vi "Main.vi"() -> ()   [LabVIEW 2020, in "Application.lvlib"]
uses:
  Application.lvlib
  Data Manager/Name--cluster.ctl
  Data Manager/Profile--cluster.ctl
  Strava/Strava curl/Strava curl.lvclass
  Data Manager/Data Manager.lvclass
  Globals.vi
  <userlib>/FTools/JSON Pretty Printer/JSON Pretty Printer.lvlib
  Twitter/Twitter.lvclass
  Visualisation/Visualisation.lvclass
panel:
  out "Status":string
  out "Errors":errorcluster[](array[cluster])
  in  "Tab":T1(tab)
  in  "Date for Daily Gains":timestamp format="%<%x %.3X>T"
  in  "Download from Strava":bool
  in  "Strava":T2={"Club ID"="RockCrusaders", "page"="1", "per_page"="200", "Authentication Token"=""}
  in  "Update Athlete":bool
  out "Athlete Profile Map":map{T3, T4}(c390)
  in  "Load Members":bool
  in  "path to PNG file":path=path "C:/Users/User/Documents/GitHub/StravaLabVIEWTwitter/Exports/To Publish.png"
  in  "Tweet":string="\n\n@RockcrusadersO #Strava #Run #Walk #Ride #FebruaryChallenge #TweetBot"
  in  "Tweet with Image":bool
  in  "Preview":bool
  out "History":string[][](table)
  in  "SQL":string
  out "Return":string[][](table)
  in  "Run SQL":bool
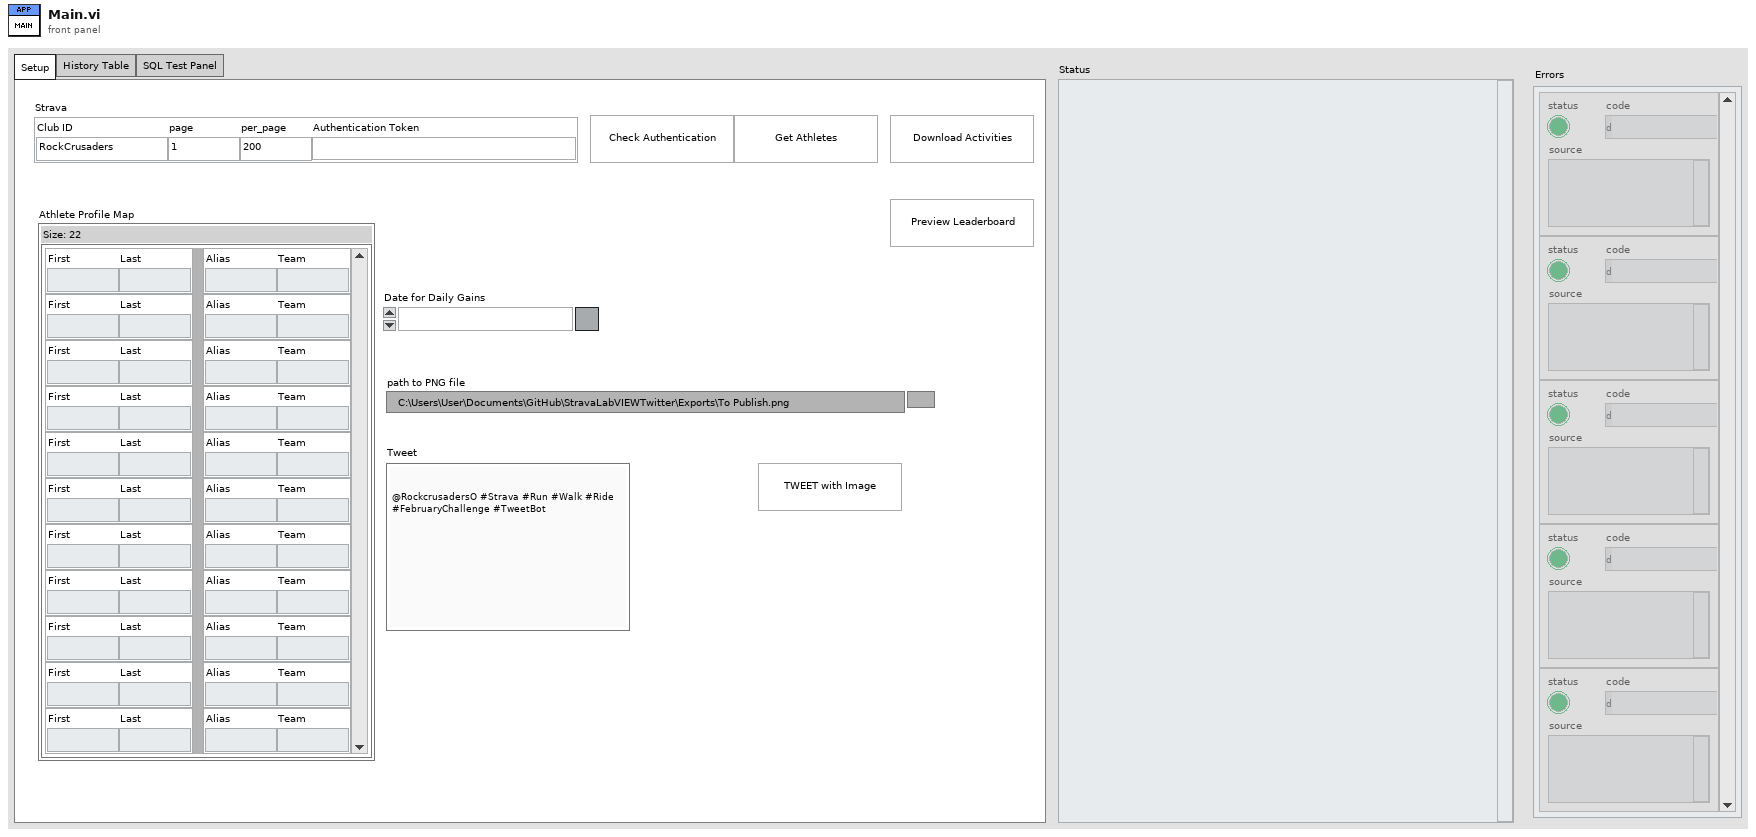
[diagram p1: front panel]
types:
  T1 = enum32{"Setup", "History Table", "SQL Test Panel"}
  T2 = cluster{"Club ID":string, "page":string, "per_page":string, "Authentication Token":string}
  T3 = typedef "Data Manager.lvclass/Name--cluster.ctl" = cluster{"First":string, "Last":string}
  T4 = typedef "Data Manager.lvclass/Profile--cluster.ctl" = cluster{"Alias":string, "Team":string}
  T5 = enum32{"Invalid", "Standard", "Closed", "Hidden", "Minimized", "Maximized"}
  T6 = enum32{"invalid app kind", "Development System", "Run Time System", "Student Edition", "Embedded LabVIEW", "Evaluation", "Custom"}
  T7 = cluster{"Record Headers":string[], "All Records":string[][]}
  T8 = cluster{"Core":cluster{"Current VI Reference":refnum<vi>, "Close Panel on Exit?":bool}, "Errors":errorcluster[], "Strava":refnum<class "Strava curl.lvclass">, "Data Manager":refnum<class "Data Manager.lvclass">}
  T9 = cluster{"Current VI Reference":refnum<vi>, "Close Panel on Exit?":bool}
  T10 = typedef "Data Manager.lvclass/Strava JSON for Club Activities--cluster.ctl" = cluster{"athlete":cluster{"firstname":string, "lastname":string}, "type":string, "distance":dbl, "moving_time":dbl, "elapsed_time":dbl, "total_elevation_gain":dbl}
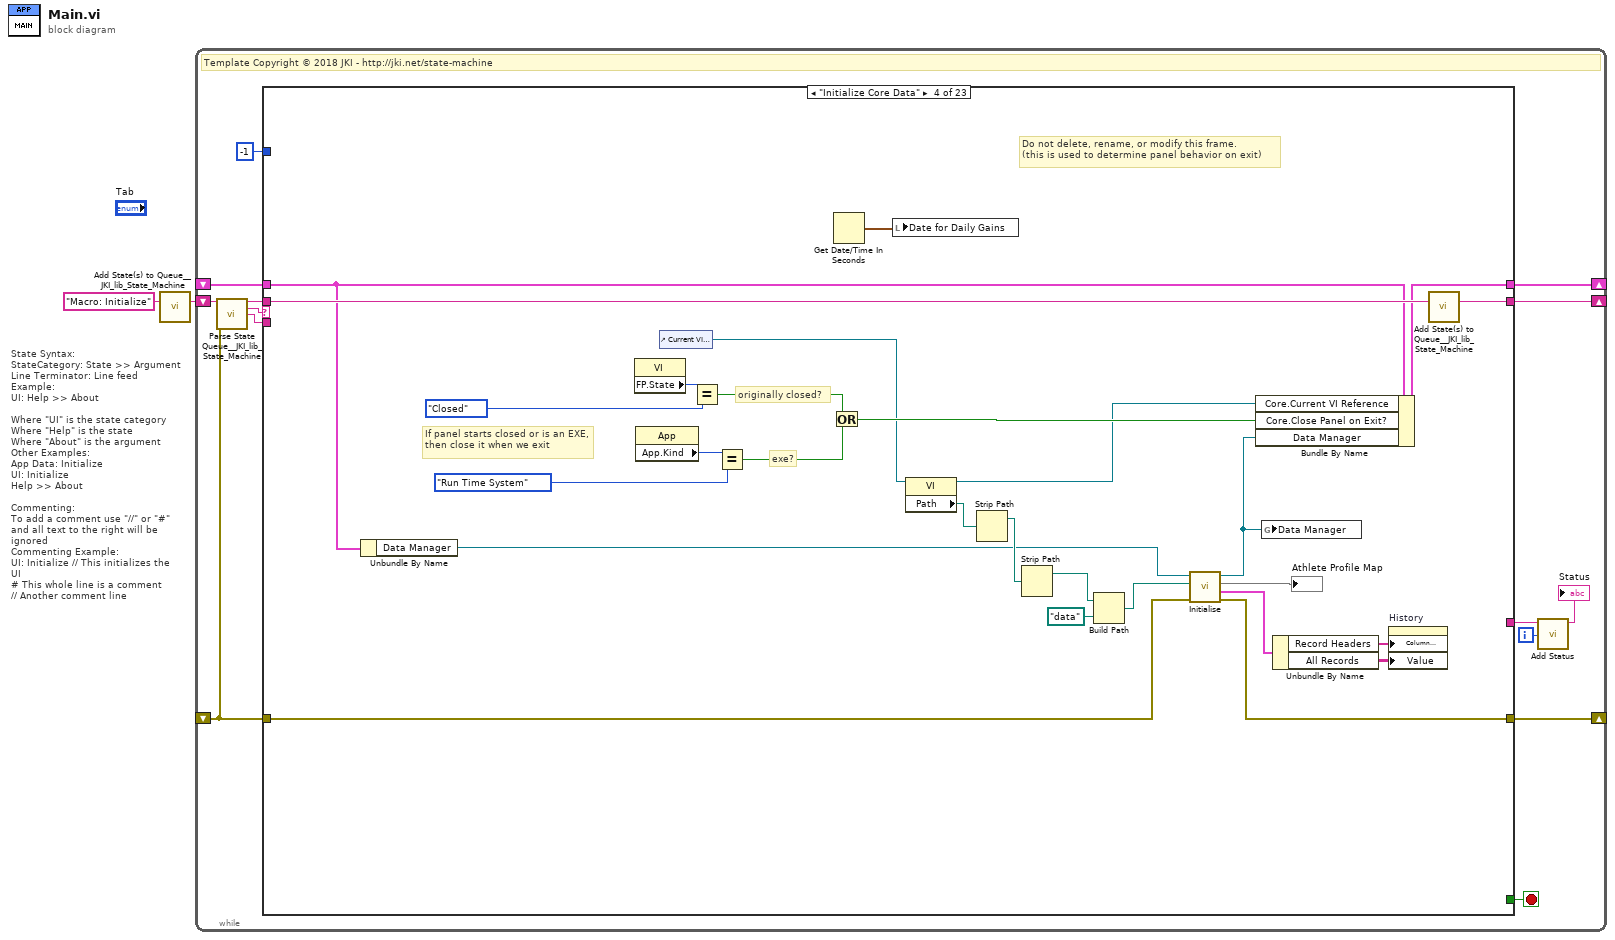
[diagram p0: block diagram]
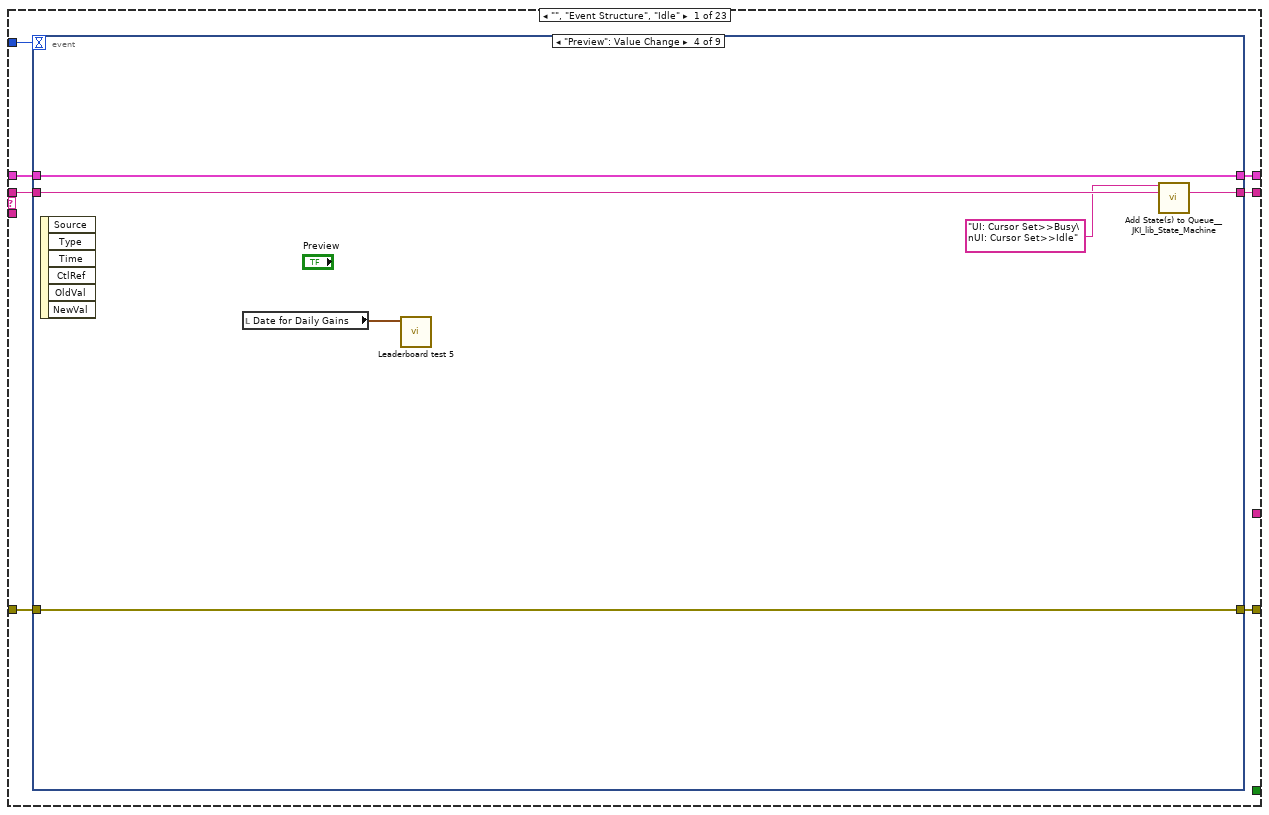
[diagram p2: hidden frame]
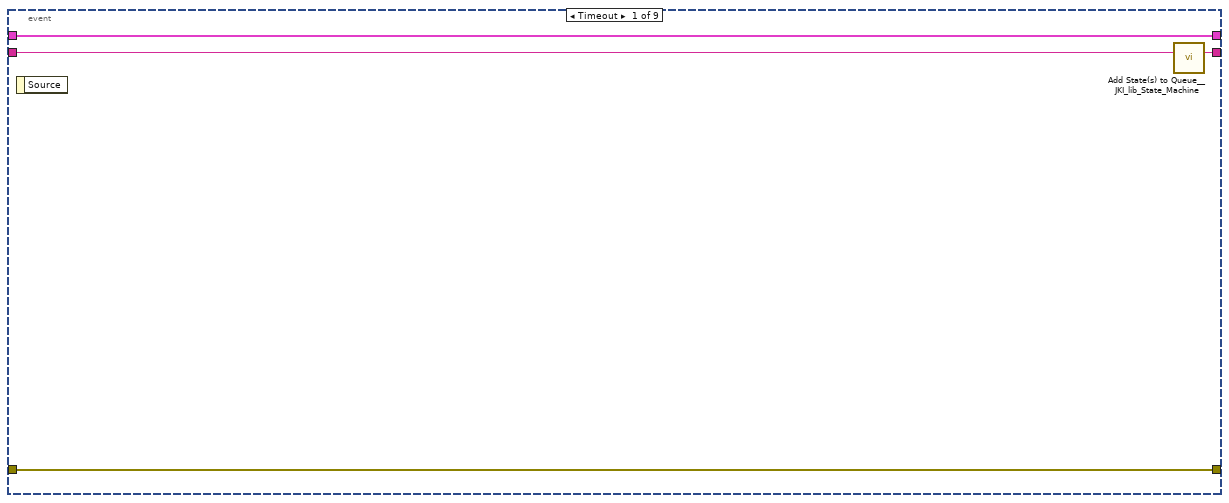
[diagram p3: hidden frame]
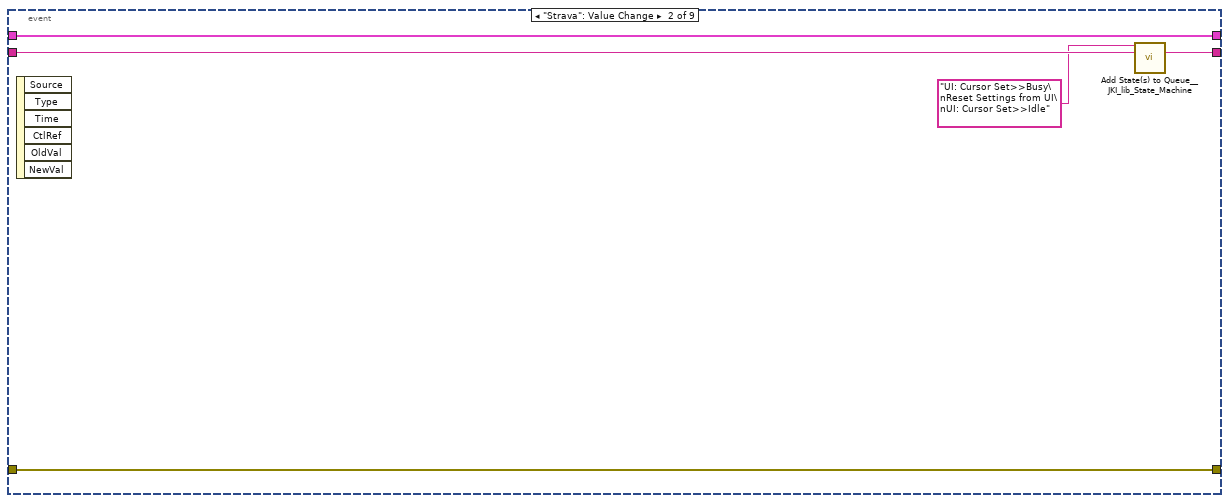
[diagram p4: hidden frame]
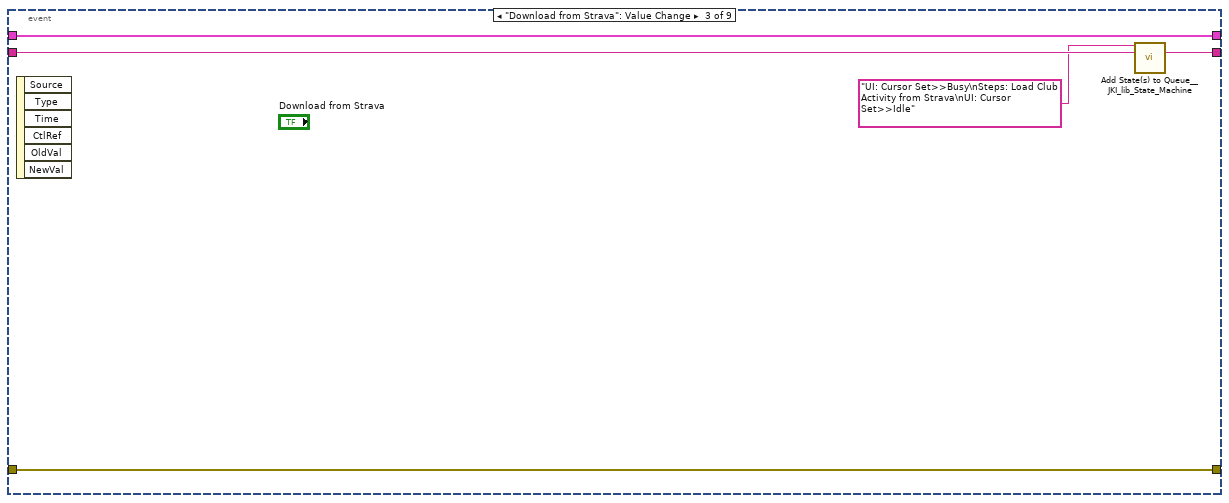
[diagram p5: hidden frame]
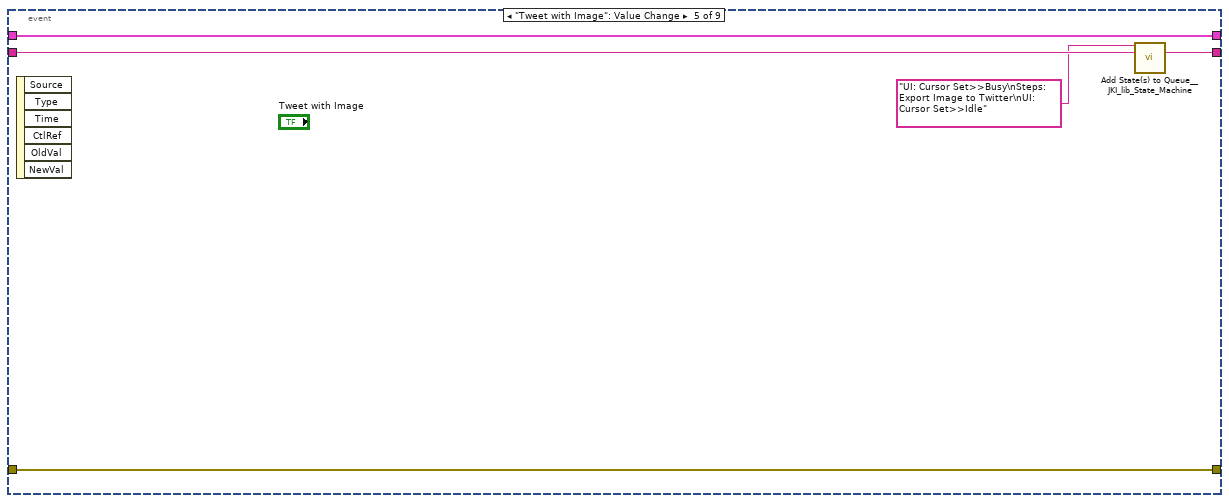
[diagram p6: hidden frame]
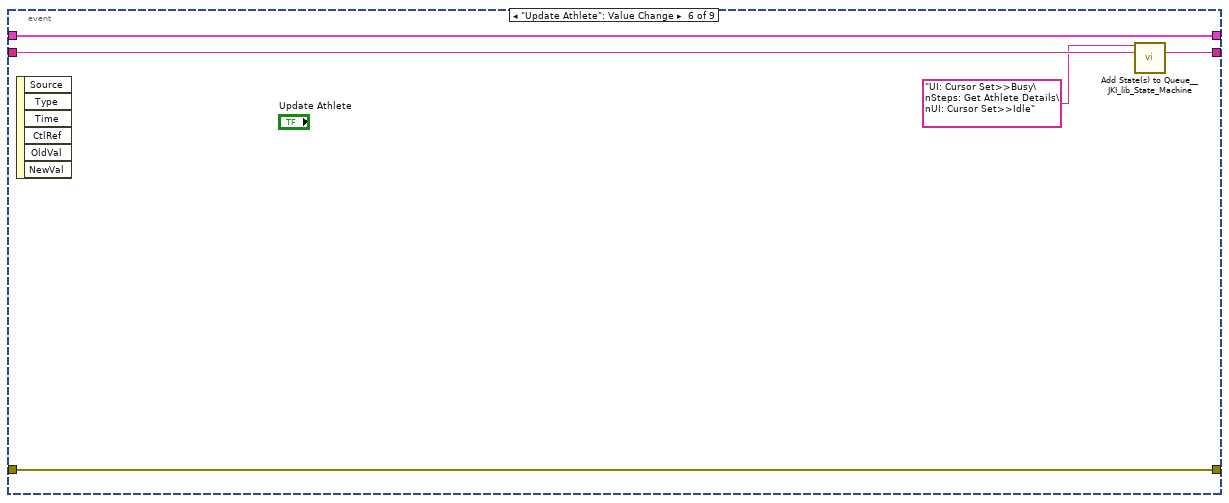
[diagram p7: hidden frame]
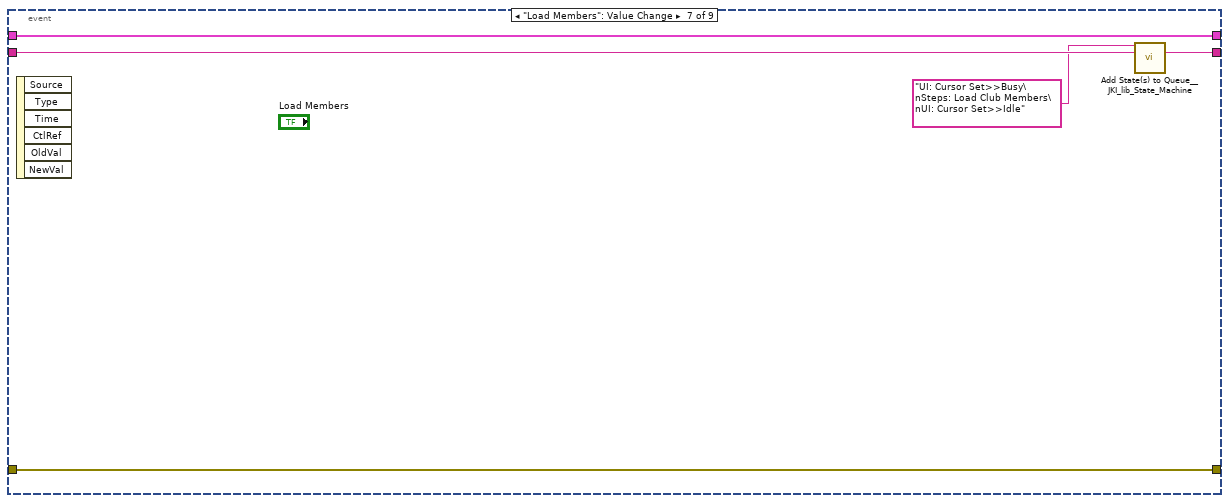
[diagram p8: hidden frame]
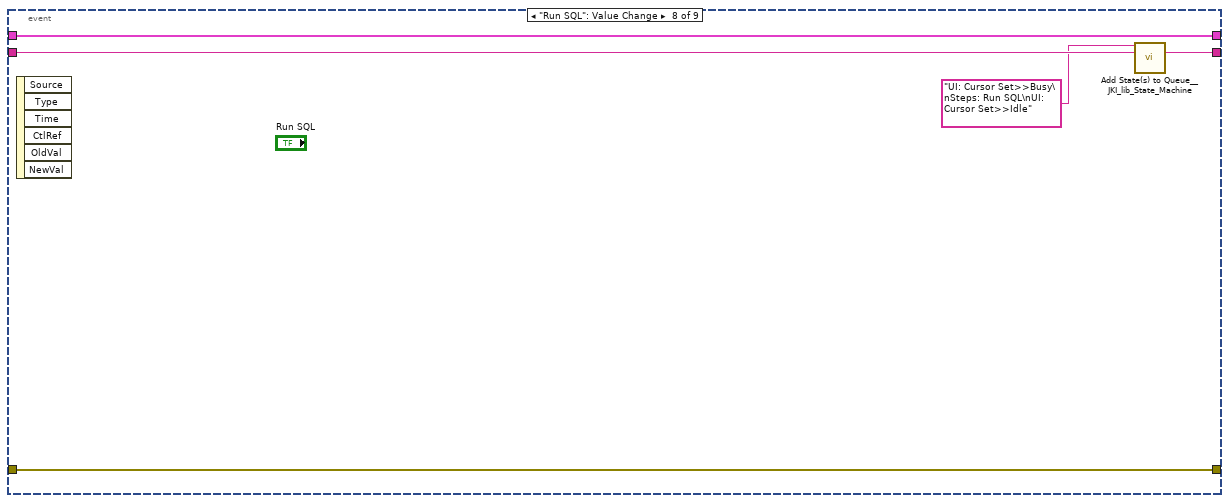
[diagram p9: hidden frame]
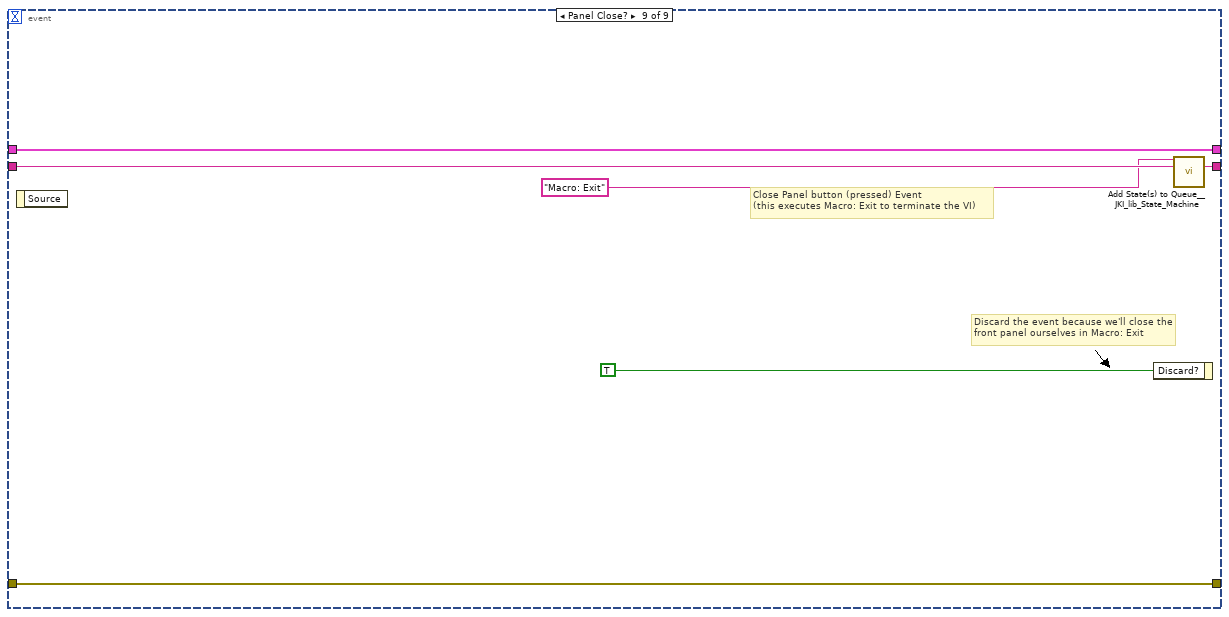
[diagram p10: hidden frame]
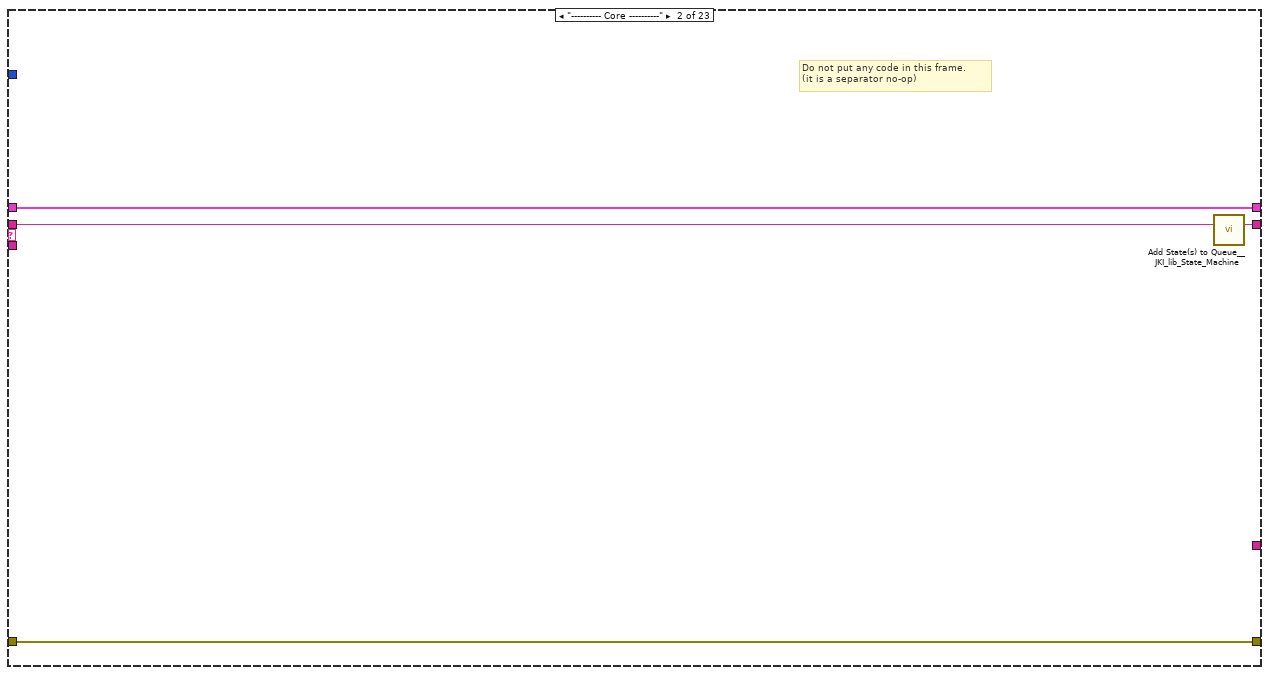
[diagram p11: hidden frame]
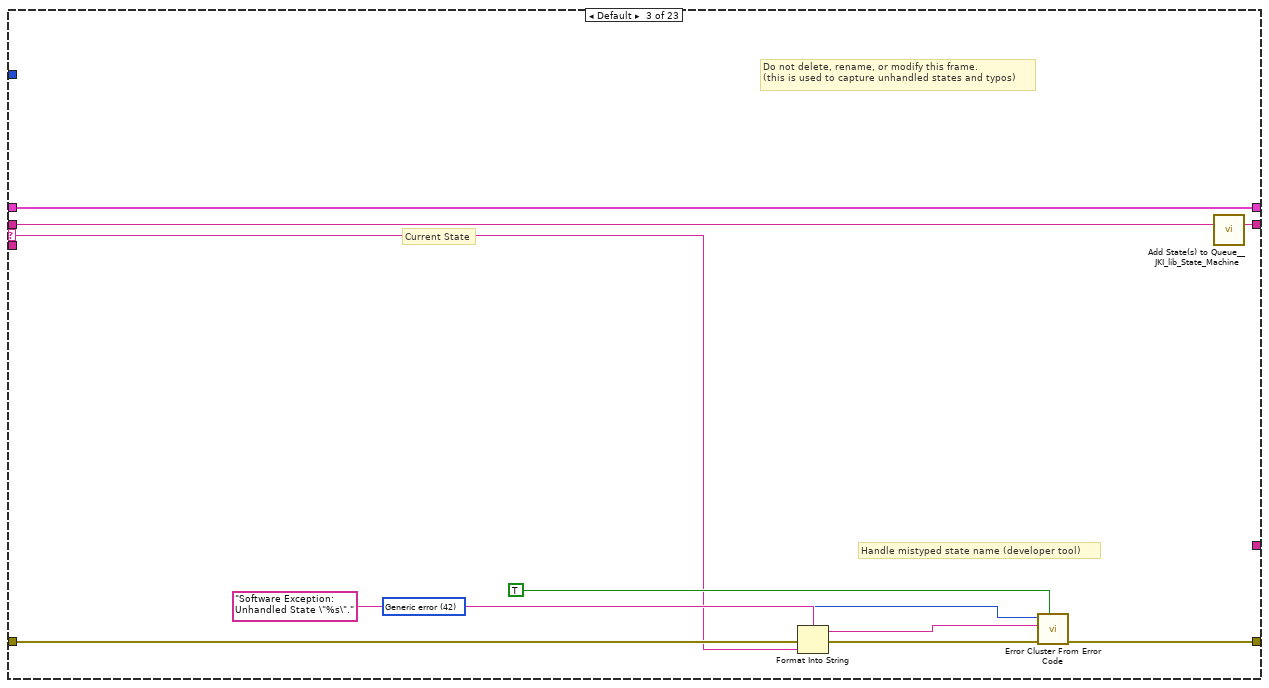
[diagram p12: hidden frame]
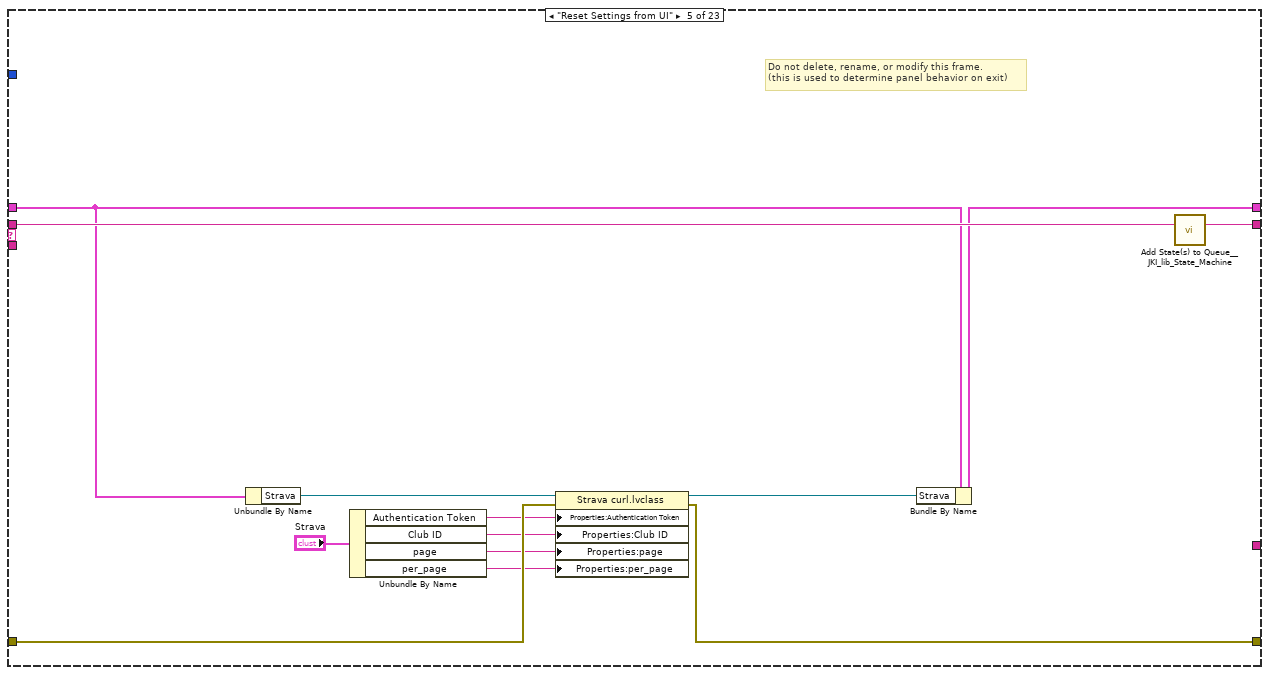
[diagram p13: hidden frame]
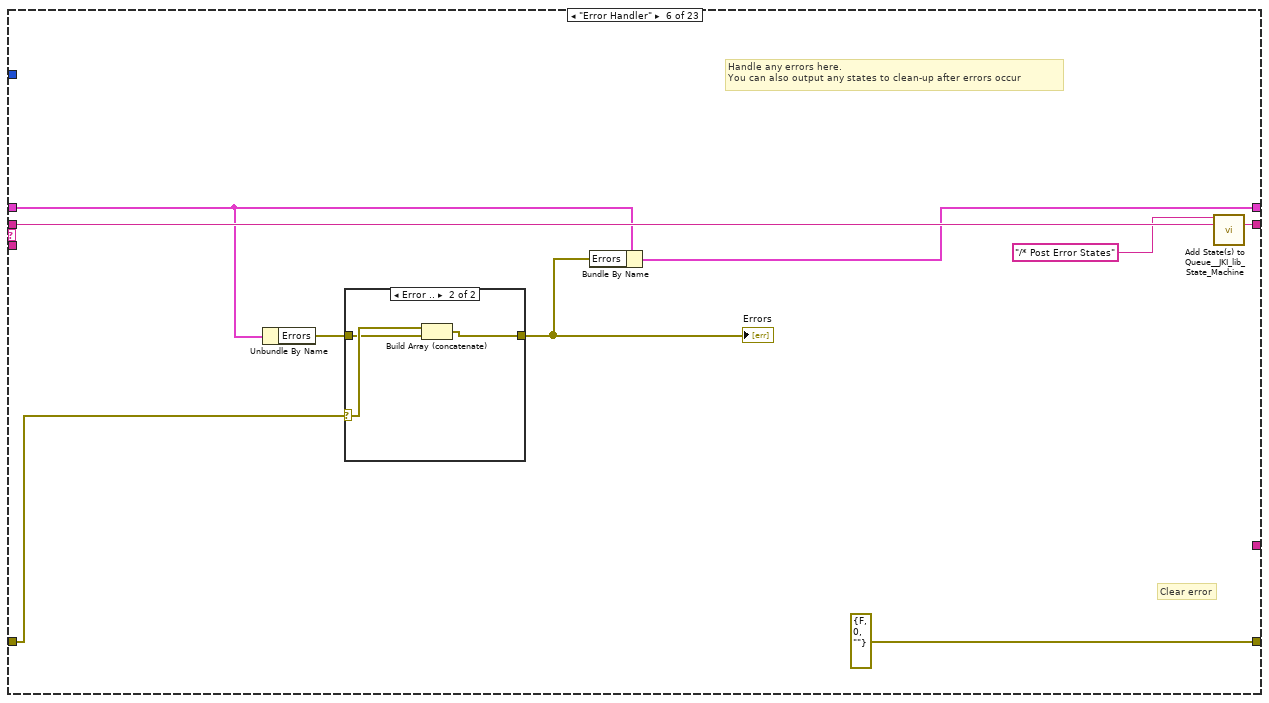
[diagram p14: hidden frame]
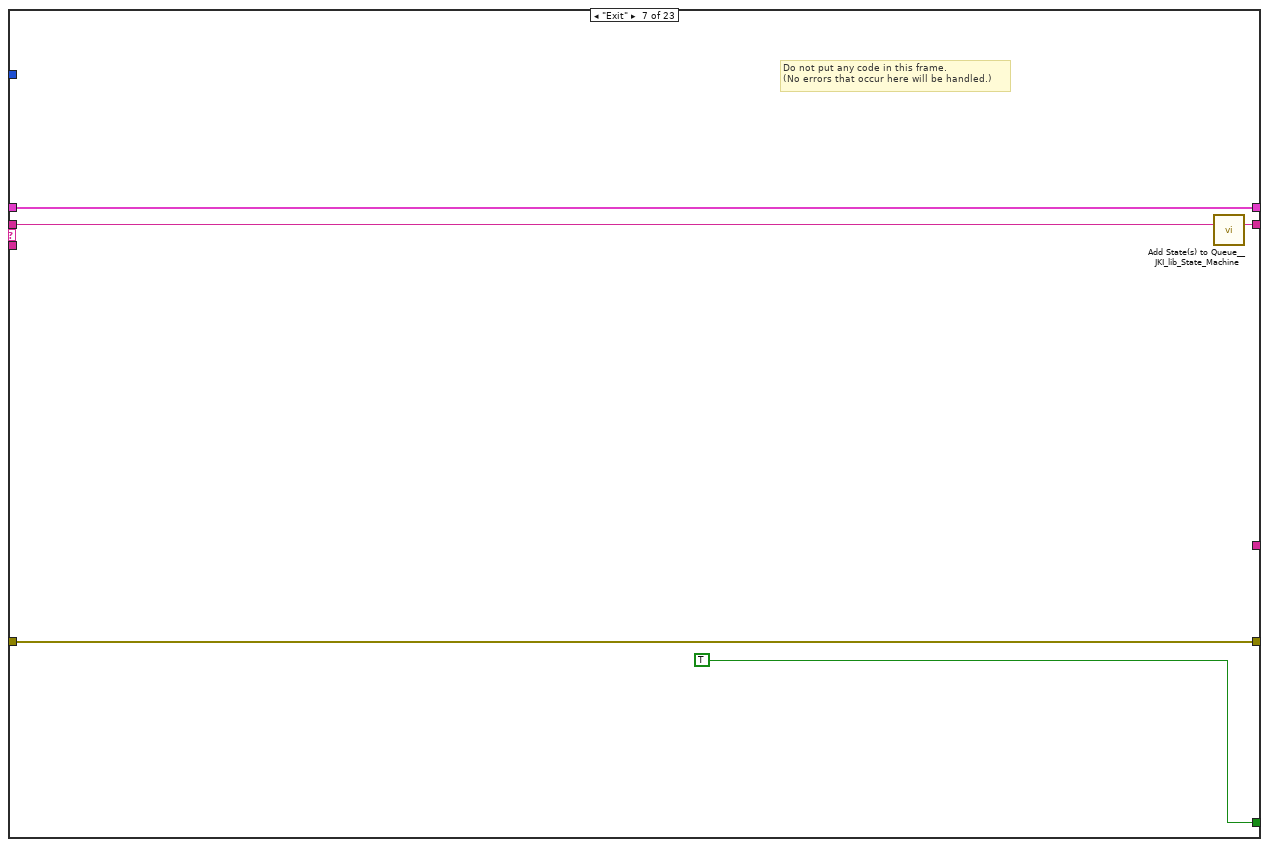
[diagram p16: hidden frame]
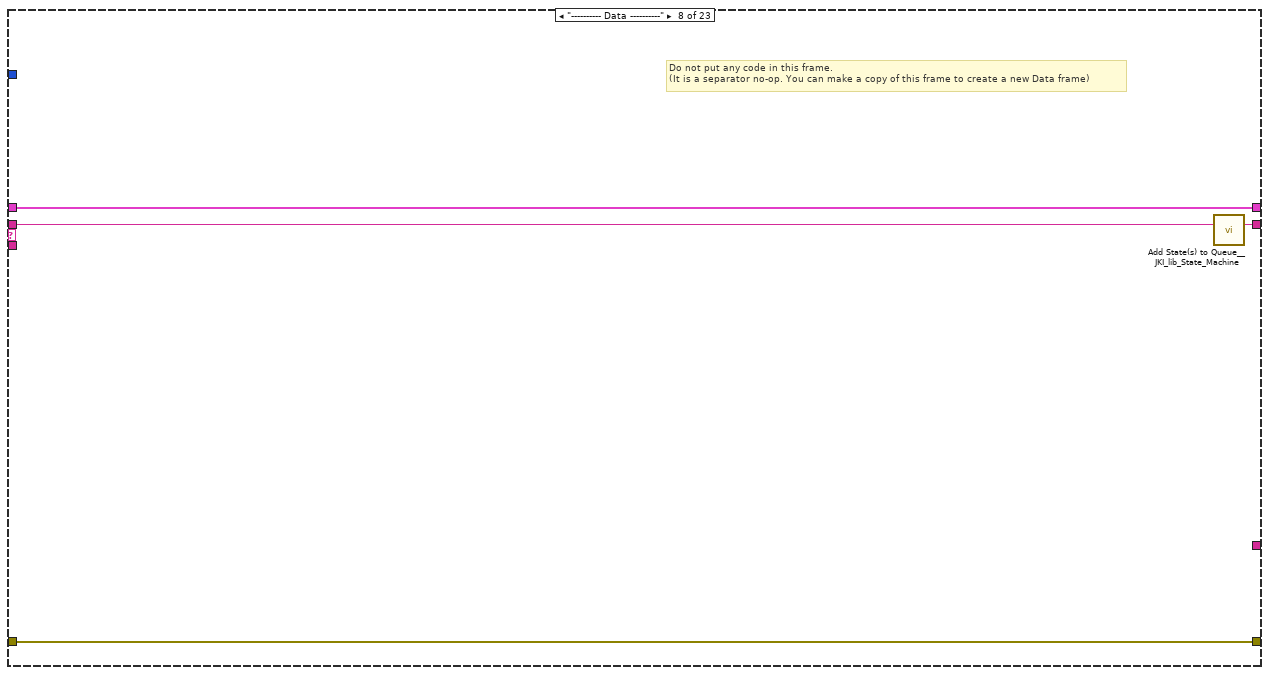
[diagram p17: hidden frame]
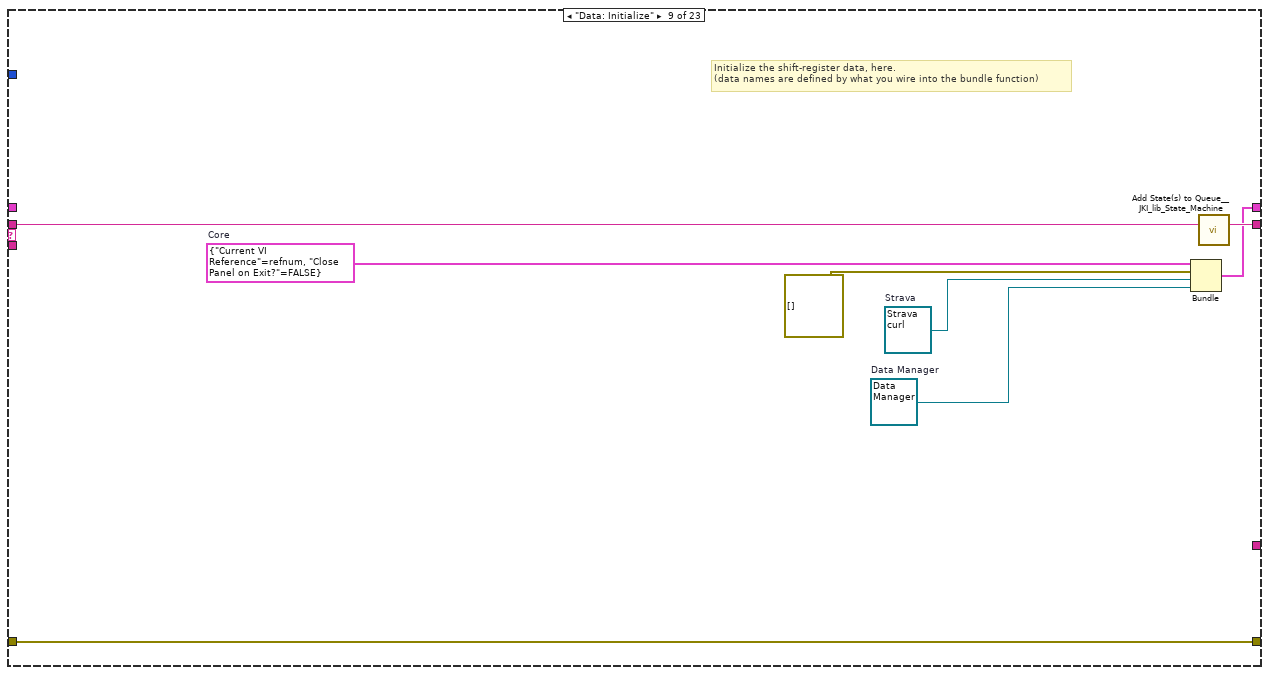
[diagram p18: hidden frame]
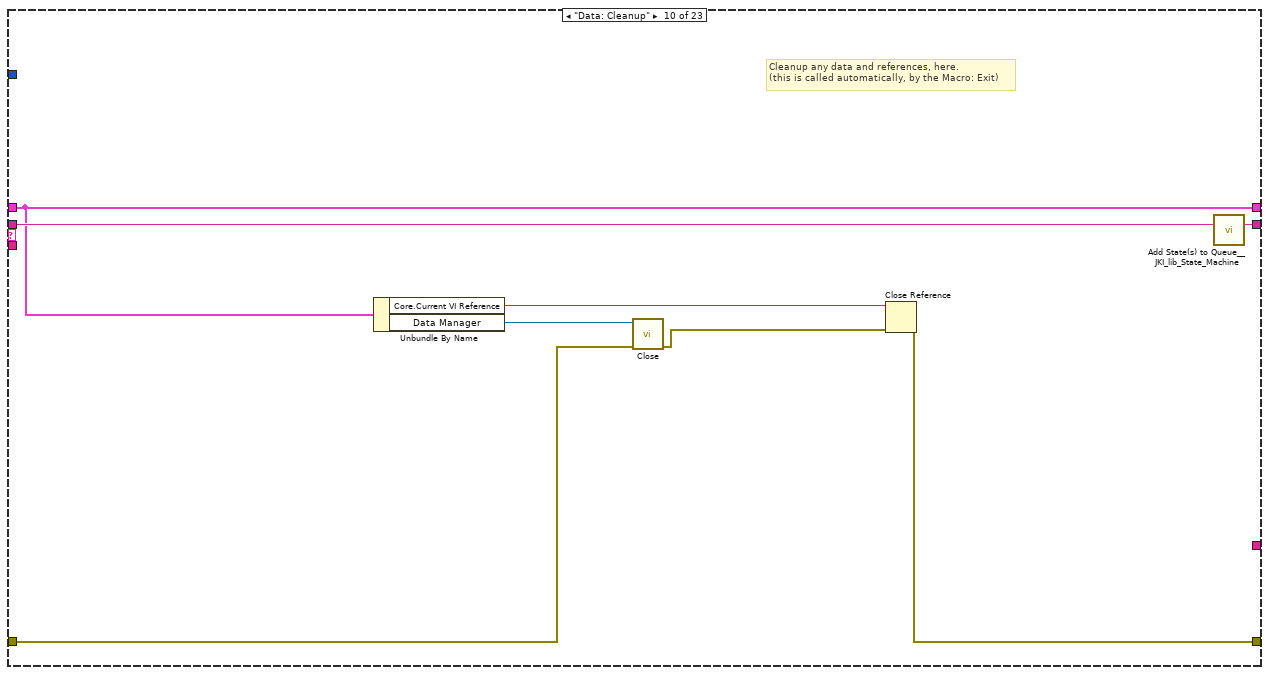
[diagram p19: hidden frame]
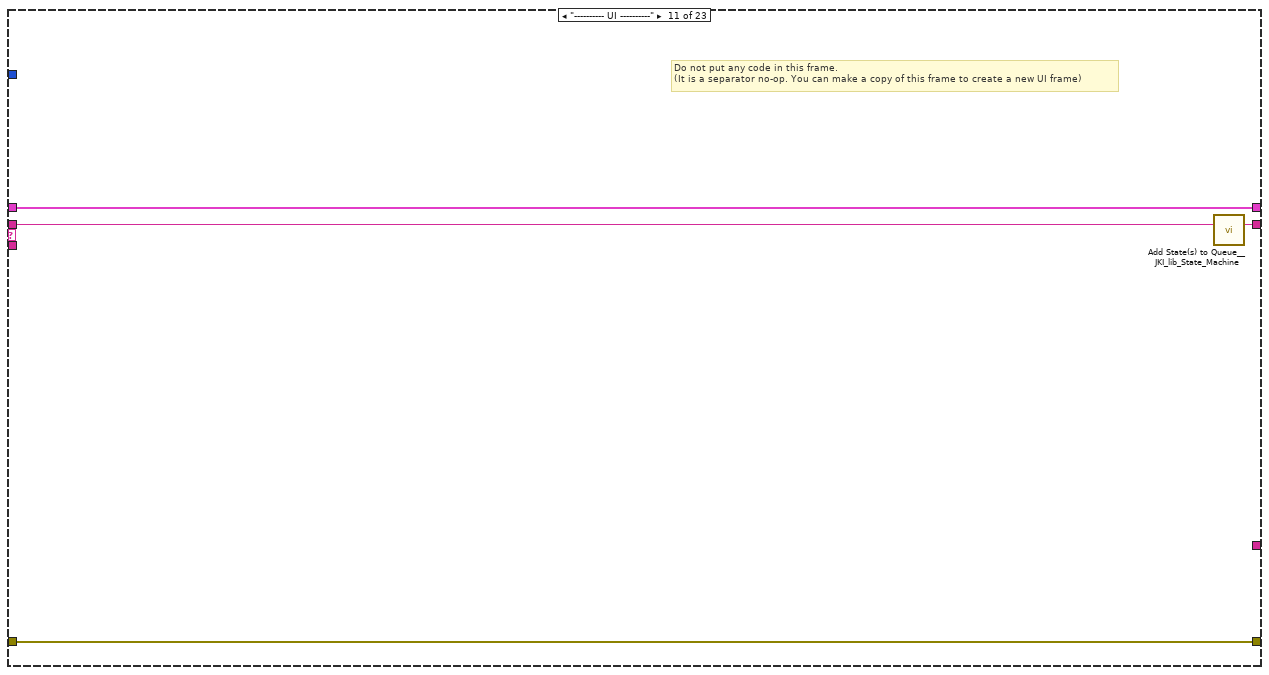
[diagram p20: hidden frame]
diagram:
  # "State Syntax:\nStateCategory: State >> Argument\nLine Terminator: Line feed\nExample:\nUI: Help >> About\n\nWhere \"UI\" is the state category\nWhere \"Help\" is the state\nWhere \"About\" is the argument\nOther Examples:\nApp Data: Initialize\nUI: Initialize\nHelp >> About\n\nCommenting:\nTo add a comment use \"//\" or \"#\" and all text to the right will be ignored\nCommenting Example:\nUI: Initialize // This initializes the UI\n# This whole line is a comment\n// Another comment line"
  n1 = call <vilib>:"Add State(s) to Queue__JKI_lib_State_Machine.vi"("State(s) in (\"\")"="Macro: Initialize") -> ("States Out"=w2:string)  [unwired: 14 in]
  n2 = while {
    shift-right: [w9] -> _
    shift-left: _ -> [w8]
    shift-right: [w12] -> _
    shift-left: _ -> [w6]
    shift-right: [w11] -> _
    shift-left: w2 -> [w13]
    i -> [w5]
    stop <- w10 stop-if-true
    # "Template Copyright © 2018 JKI - http://jki.net/state-machine"
    n3 = call <vilib>:"Parse State Queue__JKI_lib_State_Machine.vi"("State Queue"=w13, "Error In (no error)"=w6) -> ("Remaining States"=w15:string, "Current State"=w16:string, "Arguments"=w14:string)  [unwired: 11 in]
    n4 = case shown="\"Initialize Core Data\"" w16 {
      selector: w16 -> [_ _ w74 _ _ _ _ _ _ _ _ _ _ _ _ _ _ _ _ _ _ _ _]
      tunnel: w15 -> [w23 w73 w78 w111 w124 w133 w142 w146 w154 w162 w166 w170 w176 w187 w256 w261 w271 w275 w286 w307 w322 w335 w343]
      tunnel: w14 -> [_ _ _ _ _ _ _ _ _ _ _ _ w171 w181 _ _ _ _ _ _ _ _ _]
      tunnel: w8 -> [w21 w70 w76 w95 w121 w128 w140 w143 _ w158 w163 w168 w174 w183 w253 w258 w268 w272 w283 w305 w320 w333 w341]
      tunnel: [w20 w71 w80 w91 w112 errorcluster {"status"=FALSE, "code"=0, "source"=""} ("error out") w139 w144 w151 w159 w164 w167 w172 w184 w254 w259 w269 w273 w279 w301 w316 w325 w338] -> w12
      tunnel: w6 -> [w19 w71 w79 w92 w119 w125 w139 w144 w151 w156 w164 w167 w173 w185 w254 w259 w269 w273 w276 w303 w318 w329 _]
      tunnel: [w22 w72 w77 w110 w123 w132 w141 w145 w153 w161 w165 w169 w175 w186 w255 w260 w270 w274 w285 w306 w321 w334 w342] -> w11
      tunnel: [_ _ _ _ _ _ TRUE _ _ _ _ _ _ _ _ _ _ _ _ _ _ _ _] -> w10
      tunnel: [w18 w70 w76 w109 w122 w127 w140 w143 w152 w158 w163 w168 w174 w183 w253 w258 w268 w272 w284 w302 w317 w332 w341] -> w9
      tunnel: -1 ("Timeout") -> [w17 _ _ _ _ _ _ _ _ _ _ _ _ _ _ _ _ _ _ _ _ _ _]
      tunnel: [_ _ _ _ _ _ _ _ _ _ _ _ _ _ _ _ _ _ w278 w290 w315 w323 _] -> w4
      frame "", "Event Structure", "Idle" {
        n5 = event shown="[3] \"Preview\": Value Change" {
          selector: _ -> [_ _ _ _ _ _ _ _ _]
          dyn-events: _ -> [_ _ _ _ _ _ _ _ _]
          timeout: w17 -> [_ _ _ _ _ _ _ _ _]
          tunnel: w23 -> [w27 w30 w35 w41 w46 w51 w56 w61 w69]
          tunnel: [w26 w31 w36 w42 w47 w52 w57 w62 w68] -> w22
          tunnel: w21 -> [w24 w32 w37 w43 w48 w53 w58 w63 w66]
          tunnel: [w25 w28 w33 w39 w44 w49 w54 w59 w67] -> w20
          tunnel: w19 -> [w25 w28 w33 w39 w44 w49 w54 w59 w67]
          tunnel: [w24 w32 w37 w43 w48 w53 w58 w63 w66] -> w18
          event Timeout {
            n6 = event-data() -> ()  [unwired: 1 in, 1 out]
            n7 = call <vilib>:"Add State(s) to Queue__JKI_lib_State_Machine.vi"("State(s) in (\"\")"=w27) -> ("States Out"=w26:string)  [unwired: 14 in]
          }
          event "Strava": Value Change {
            n8 = event-data() -> ()  [unwired: 1 in, 6 out]
            n9 = call <vilib>:"Add State(s) to Queue__JKI_lib_State_Machine.vi"("State(s) in Front (\"\")"="UI: Cursor Set>>Busy\nReset Settings from UI\nUI: Cursor Set>>Idle" ("State(s) in Front (\"\")"), "State(s) in (\"\")"=w30) -> ("States Out"=w31:string)  [unwired: 13 in]
          }
          event "Download from Strava": Value Change {
            n10 = event-data() -> ()  [unwired: 1 in, 6 out]
            n11 = call <vilib>:"Add State(s) to Queue__JKI_lib_State_Machine.vi"("State(s) in Front (\"\")"="UI: Cursor Set>>Busy\nSteps: Load Club Activity from Strava\nUI: Cursor Set>>Idle" ("State(s) in Front (\"\")"), "State(s) in (\"\")"=w35) -> ("States Out"=w36:string)  [unwired: 13 in]
          }
          event "Preview": Value Change {
            n12 = event-data() -> ()  [unwired: 1 in, 6 out]
            n13 = local read "Date for Daily Gains"() -> (w38:timestamp)
            n14 = call "Leaderboard test 5.vi"("current time"=w38) -> ()  [unwired: 11 in]
            n15 = call <vilib>:"Add State(s) to Queue__JKI_lib_State_Machine.vi"("State(s) in Front (\"\")"="UI: Cursor Set>>Busy\nUI: Cursor Set>>Idle" ("State(s) in Front (\"\")"), "State(s) in (\"\")"=w41) -> ("States Out"=w42:string)  [unwired: 13 in]
          }
          event "Tweet with Image": Value Change {
            n16 = event-data() -> ()  [unwired: 1 in, 6 out]
            n17 = call <vilib>:"Add State(s) to Queue__JKI_lib_State_Machine.vi"("State(s) in Front (\"\")"="UI: Cursor Set>>Busy\nSteps: Export Image to Twitter\nUI: Cursor Set>>Idle" ("State(s) in Front (\"\")"), "State(s) in (\"\")"=w46) -> ("States Out"=w47:string)  [unwired: 13 in]
          }
          event "Update Athlete": Value Change {
            n18 = event-data() -> ()  [unwired: 1 in, 6 out]
            n19 = call <vilib>:"Add State(s) to Queue__JKI_lib_State_Machine.vi"("State(s) in Front (\"\")"="UI: Cursor Set>>Busy\nSteps: Get Athlete Details\nUI: Cursor Set>>Idle" ("State(s) in Front (\"\")"), "State(s) in (\"\")"=w51) -> ("States Out"=w52:string)  [unwired: 13 in]
          }
          event "Load Members": Value Change {
            n20 = event-data() -> ()  [unwired: 1 in, 6 out]
            n21 = call <vilib>:"Add State(s) to Queue__JKI_lib_State_Machine.vi"("State(s) in Front (\"\")"="UI: Cursor Set>>Busy\nSteps: Load Club Members\nUI: Cursor Set>>Idle" ("State(s) in Front (\"\")"), "State(s) in (\"\")"=w56) -> ("States Out"=w57:string)  [unwired: 13 in]
          }
          event "Run SQL": Value Change {
            n22 = event-data() -> ()  [unwired: 1 in, 6 out]
            n23 = call <vilib>:"Add State(s) to Queue__JKI_lib_State_Machine.vi"("State(s) in Front (\"\")"="UI: Cursor Set>>Busy\nSteps: Run SQL\nUI: Cursor Set>>Idle" ("State(s) in Front (\"\")"), "State(s) in (\"\")"=w61) -> ("States Out"=w62:string)  [unwired: 13 in]
          }
          event Panel Close? {
            # "Discard the event because we'll close the front panel ourselves in Macro: Exit"
            # "Close Panel button (pressed) Event\n(this executes Macro: Exit to terminate the VI)"
            n24 = event-data() -> ()  [unwired: 1 in, 1 out]
            n25 = event-data("Discard?"=TRUE) -> ()  [unwired: 1 in, 1 out]
            n26 = call <vilib>:"Add State(s) to Queue__JKI_lib_State_Machine.vi"("State(s) in Front (\"\")"="Macro: Exit", "State(s) in (\"\")"=w69) -> ("States Out"=w68:string)  [unwired: 13 in]
          }
        }
      }
      frame "---------- Core ----------" {
        # "Do not put any code in this frame.\n(it is a separator no-op)"
        n27 = call <vilib>:"Add State(s) to Queue__JKI_lib_State_Machine.vi"("State(s) in (\"\")"=w73) -> ("States Out"=w72:string)  [unwired: 14 in]
      }
      frame Default {
        w83 = 42 items=["No error", "Argument error", "Memory is full", "Out of zone", "End of file", "File already open", "Generic file I/O error", "File not found", "File permission error", "Disk is full", "Duplicate path", "Too many files open", "System feature not enabled", "Resource file not found", "Cannot add resource", "Resource not found", "Image not found", "Image memory error", "Pen does not exist", "Config type invalid", "Config token not found", "Config parse error", "Config memory error", "Bad external code format", "Bad external code offset", "External code not present", "Null window", "Destroy window error", "Null menu", "Print aborted", "Bad print record", "Print driver error", "Windows error during printing", "Memory error during printing", "Print dialog error", "Generic print error", "Invalid device refnum", "Device not found", "Device parameter error", "Device unit error", "Cannot open device", "Device call aborted", "Generic error", "Cancelled by user", "Object ID too low", "Object ID too high", "Object not in heap", "Unknown heap", "Unknown object (invalid DefProc)", "Unknown object (DefProc not in table)", "Message out of range", "Invalid (null) method", "Unknown message", "Manager call not supported", "Bad address", "Network operation in progress", "Network operation timed out", "Connection is busy", "Network attribute not supported", "Network error", "Address in use", "System out of memory", "Connection aborted", "Connection refused", "Not connected", "Already connected", "Connection closed", "Initialization error (interapplication manager)", "Bad occurrence", "Wait on unbound occurrence handler", "Occurrence queue overflow", "Datalog type conflict", "Unused", "Unrecognized type (interapplication manager)", "Memory corrupt", "Failed to make temporary DLL", "Old CIN version", "Drag socket not found", "Failed to load drop-object", "Failed to register OLE object", "Failed to release OLE object", "Format specifier type mismatch", "Unknown format specifier", "Too few format specifiers", "Too many format specifiers", "Scan failed", "Newer CIN version", "Error converting to variant", "Runtime menu error", "Password tampered", "Variant attribute not found", "Incompatible variant data type", "Event data is not available", "Event Store is not present", "Occurrence is not found", "Event Queue is not created", "Event info is not available", "Refnum passed is NULL", "Error retrieving Class GUID", "Error retrieving CoClass GUID", "Error retrieving TypeLib GUID.", "Bad built application magic bytes.", "Specific driver is different from the specific driver associated with the Logical Name.", "There is no session opened to the class driver.", "Max Error", "MAX - Error with config objects", "MAX - Error loading configuration", "MAX - Group not supported"]
        # "Current State"
        # "Do not delete, rename, or modify this frame.\n(this is used to capture unhandled states and typos)"
        # "Handle mistyped state name (developer tool)"
        n28 = Format Into String(format string="Software Exception: Unhandled State \"%s\"." ("message"), error in=w79, w74) -> (resulting string=w82:string, error out=w81:errorcluster)  [unwired: 1 in]
        n29 = call <vilib>:"Error Cluster From Error Code.vi"("show call chain? (False)"=TRUE, "error in (no error)"=w81, "error message (\"\")"=w82, "error code (0)"=w83) -> ("error out"=w80:errorcluster)  [unwired: 5 in]
        n30 = call <vilib>:"Add State(s) to Queue__JKI_lib_State_Machine.vi"("State(s) in (\"\")"=w78) -> ("States Out"=w77:string)  [unwired: 14 in]
      }
      frame "Initialize Core Data" {
        # "Do not delete, rename, or modify this frame.\n(this is used to determine panel behavior on exit)"
        # "originally closed?"
        # "exe?"
        # "If panel starts closed or is an EXE, then close it when we exit"
        n31 = Unbundle By Name(w95) -> ("Data Manager"=w94:refnum<class "Data Manager.lvclass">)
        n32 = property class="VI"() -> ("FP.State"=w104:T5)  [unwired: 2 in, 2 out]
        n33 = property class="App"() -> ("App.Kind"=w108:T6)  [unwired: 2 in, 2 out]
        n34 = control-ref of="Current VI Reference"() -> (w101:refnum<vi>)
        n35 = Equal?(x=w104, y=T5."Closed" ("Front Panel Window:State")) -> (x = y?=w102:bool)
        n36 = Equal?(x=w108, y=T6."Run Time System" ("Application:Kind")) -> (x = y?=w106:bool)
        n37 = Or(x=w102, y=w106) -> (x .or. y?=w105:bool)
        n38 = Get Date/Time In Seconds() -> (seconds since 1Jan1904=w85:timestamp)
        n39 = local write "Date for Daily Gains"(w85) -> ()
        n40 = property class="VI"(reference=w101) -> (reference out=w100:refnum<vi>, "Path"=w99:path)  [unwired: 1 in, 1 out]
        n41 = Strip Path(path=w99) -> (stripped path=w98:path)  [unwired: 1 out]
        n42 = Strip Path(path=w98) -> (stripped path=w97:path)  [unwired: 1 out]
        n43 = Build Path(base path=w97, name or relative path=path "data") -> (appended path=w93:path)
        n44 = call-dynamic "Initialise.vi"("error in (no error)"=w92, "Data Folder"=w93, "Data Manager in"=w94) -> ("error out"=w91:errorcluster, "History"=w89:T7, "Athlete Profile Map"=→"Athlete Profile Map":map{T3, T4}, "Data Manager out"=w86:refnum<class "Data Manager.lvclass">)  [unwired: 5 in]
        n45 = Bundle By Name(cluster=w95, "Core.Current VI Reference"=w100, "Core.Close Panel on Exit?"=w105, "Data Manager"=w86) -> (w109:T8)
        n46 = global write "Globals.vi" "Data Manager"(w86) -> ()
        n47 = Unbundle By Name(w89) -> ("Record Headers"=w88:string[], "All Records"=w87:string[][])
        n48 = property on="History" class="Tbl (strict)"("Column Headers[]"=w88, "Value"=w87) -> ()  [unwired: 2 in, 2 out]
        n49 = call <vilib>:"Add State(s) to Queue__JKI_lib_State_Machine.vi"("State(s) in (\"\")"=w111) -> ("States Out"=w110:string)  [unwired: 14 in]
      }
      frame "Reset Settings from UI" {
        # "Do not delete, rename, or modify this frame.\n(this is used to determine panel behavior on exit)"
        n50 = Unbundle By Name(w121) -> ("Strava"=w120:refnum<class "Strava curl.lvclass">)
        n51 = Unbundle By Name("Strava") -> ("Authentication Token"=w115:string, "Club ID"=w118:string, "page"=w117:string, "per_page"=w116:string)
        n52 = property class="Strava curl.lvclass"(reference=w120, error in=w119, "Properties:Authentication Token"=w115, "Properties:Club ID"=w118, "Properties:page"=w117, "Properties:per_page"=w116) -> (reference out=w113:refnum<class "Strava curl.lvclass">, error out=w112:errorcluster)
        n53 = Bundle By Name(cluster=w121, "Strava"=w113) -> (w122:T8)
        n54 = call <vilib>:"Add State(s) to Queue__JKI_lib_State_Machine.vi"("State(s) in (\"\")"=w124) -> ("States Out"=w123:string)  [unwired: 14 in]
      }
      frame "Error Handler" {
        # "Handle any errors here.\nYou can also output any states to clean-up after errors occur"
        # "Clear error"
        n55 = Unbundle By Name(w128) -> ("Errors"=w129:errorcluster[])
        n56 = case shown="Error .." w125 {
          selector: w125 -> [_ w137]
          tunnel: w129 -> [w134 w136]
          tunnel: [w134 w135] -> w126
          frame No Error {
          }
          frame Error {
            n57 = Build Array (concatenate)(w137, w136) -> (w135:errorcluster[])
          }
        }
        "Errors" <- w126
        n58 = Bundle By Name(cluster=w128, "Errors"=w126) -> (w127:T8)
        n59 = call <vilib>:"Add State(s) to Queue__JKI_lib_State_Machine.vi"("State(s) in Front (\"\")"="/* Post Error States", "State(s) in (\"\")"=w133) -> ("States Out"=w132:string)  [unwired: 13 in]
      }
      frame "Exit" {
        # "Do not put any code in this frame.\n(No errors that occur here will be handled.)"
        n60 = call <vilib>:"Add State(s) to Queue__JKI_lib_State_Machine.vi"("State(s) in (\"\")"=w142) -> ("States Out"=w141:string)  [unwired: 14 in]
      }
      frame "---------- Data ----------" {
        # "Do not put any code in this frame.\n(It is a separator no-op. You can make a copy of this frame to create a new Data frame)"
        n61 = call <vilib>:"Add State(s) to Queue__JKI_lib_State_Machine.vi"("State(s) in (\"\")"=w146) -> ("States Out"=w145:string)  [unwired: 14 in]
      }
      frame "Data: Initialize" {
        w147 = refnum<class "Data Manager.lvclass"> refnum  # Data Manager
        w148 = refnum<class "Strava curl.lvclass"> refnum  # Strava
        w150 = T9 {"Current VI Reference"=refnum, "Close Panel on Exit?"=FALSE}  # Core
        # "Initialize the shift-register data, here.\n(data names are defined by what you wire into the bundle function)"
        n62 = Bundle("Core"=w150, "Errors"=errorcluster[] [], "Strava"=w148, "Data Manager"=w147) -> (w152:T8)  [unwired: 1 in]
        n63 = call <vilib>:"Add State(s) to Queue__JKI_lib_State_Machine.vi"("State(s) in (\"\")"=w154) -> ("States Out"=w153:string)  [unwired: 14 in]
      }
      frame "Data: Cleanup" {
        # "Cleanup any data and references, here.\n(this is called automatically, by the Macro: Exit)"
        n64 = Unbundle By Name(w158) -> ("Core.Current VI Reference"=w160:refnum<vi>, "Data Manager"=w157:refnum<class "Data Manager.lvclass">)
        n65 = call-dynamic "Close.vi"("error in (no error)"=w156, "Data Manager in"=w157) -> ("error out"=w155:errorcluster)  [unwired: 8 in, 1 out]
        n66 = Close Reference(reference=w160, error in (no error)=w155) -> (error out=w159:errorcluster)
        n67 = call <vilib>:"Add State(s) to Queue__JKI_lib_State_Machine.vi"("State(s) in (\"\")"=w162) -> ("States Out"=w161:string)  [unwired: 14 in]
      }
      frame "---------- UI ----------" {
        # "Do not put any code in this frame.\n(It is a separator no-op. You can make a copy of this frame to create a new UI frame)"
        n68 = call <vilib>:"Add State(s) to Queue__JKI_lib_State_Machine.vi"("State(s) in (\"\")"=w166) -> ("States Out"=w165:string)  [unwired: 14 in]
      }
      frame "UI: Initialize" {
        # "Initialize the User Interface, here.\n(this is called automatically, by the Macro: Init)"
        n69 = call <vilib>:"Add State(s) to Queue__JKI_lib_State_Machine.vi"("State(s) in (\"\")"=w170) -> ("States Out"=w169:string)  [unwired: 14 in]
      }
      frame "UI: Cursor Set" {
        # "Argument"
        # "Set and Unset Cursor Busy.\n(Usage: \"UI: Cursor Set >> Busy|Idle\")"
        n70 = case shown="\"Idle\", Default" w171 {
          tunnel: w173 -> [w178 w180]
          tunnel: [w177 w179] -> w172
          frame "Idle", Default {
            n71 = call <vilib>:"Unset Busy.vi"("error in (no error)"=w178) -> ("error out"=w177:errorcluster)  [unwired: 10 in]
          }
          frame "Busy" {
            n72 = call <vilib>:"Set Busy.vi"("error in (no error)"=w180) -> ("error out"=w179:errorcluster)  [unwired: 9 in, 1 out]
          }
        }
        n73 = call <vilib>:"Add State(s) to Queue__JKI_lib_State_Machine.vi"("State(s) in (\"\")"=w176) -> ("States Out"=w175:string)  [unwired: 14 in]
      }
      frame "UI: Front Panel State" {
        # "Argument"
        # "Set Front Panel Open or Closed\n(Usage: \"UI: Front Panel State >> Open|Close\")"
        n74 = Unbundle By Name(w183) -> ("Core.Current VI Reference"=w182:refnum<vi>)
        n75 = case shown="\"Minimize\", \"Minimized\"" w181 {
          tunnel: w185 -> [w193 w208 w219 w232 w245]
          tunnel: [w195 w209 w221 w234 w247] -> w184
          tunnel: w182 -> [w194 w206 w220 w233 w246]
          frame "Open", "Standard", Default {
            w188 = T5."Standard" ("State")
            n76 = property class="VI"(reference=w194, error in=w193) -> (reference out=w191:refnum<vi>, error out=w192:errorcluster, "FP.State"=w190:T5)
            n77 = Not Equal?(x=w190, y=w188) -> (x != y?=w189:bool)
            n78 = case shown="True" w189 {
              tunnel: [w199 w201] -> w195
              tunnel: w192 -> [w198 w201]
              tunnel: w191 -> [w197 _]
              tunnel: w188 -> [w196 _]
              frame True {
                n79 = invoke class="VI" method="FP.Open"(reference=w197, error in=w198, "Activate"=TRUE, "State"=w196) -> (error out=w199:errorcluster)  [unwired: 1 in, 4 out]
              }
              frame False {
              }
            }
          }
          frame "Close", "Closed" {
            n80 = property class="VI"(reference=w206, error in=w208) -> (reference out=w205:refnum<vi>, error out=w207:errorcluster, "FP.State"=w203:T5)
            n81 = Not Equal?(x=w203, y=T5."Closed" ("Front Panel Window:State")) -> (x != y?=w202:bool)
            n82 = case shown="True" w202 {
              tunnel: [w210 w213] -> w209
              tunnel: w207 -> [w210 w212]
              tunnel: w205 -> [_ w211]
              frame False {
              }
              frame True {
                n83 = invoke class="VI" method="FP.Close"(reference=w211, error in=w212) -> (error out=w213:errorcluster)  [unwired: 1 in, 2 out]
              }
            }
          }
          frame "Hidden", "Hide" {
            w214 = T5."Hidden" ("State")
            n84 = property class="VI"(reference=w220, error in=w219) -> (reference out=w217:refnum<vi>, error out=w218:errorcluster, "FP.State"=w216:T5)
            n85 = Not Equal?(x=w216, y=w214) -> (x != y?=w215:bool)
            n86 = case shown="True" w215 {
              tunnel: [w225 w226] -> w221
              tunnel: w218 -> [w224 w226]
              tunnel: w217 -> [w223 _]
              tunnel: w214 -> [w222 _]
              frame True {
                n87 = invoke class="VI" method="FP.Open"(reference=w223, error in=w224, "State"=w222) -> (error out=w225:errorcluster)  [unwired: 2 in, 4 out]
              }
              frame False {
              }
            }
          }
          frame "Minimize", "Minimized" {
            w227 = T5."Minimized" ("State")
            n88 = property class="VI"(reference=w233, error in=w232) -> (reference out=w230:refnum<vi>, error out=w231:errorcluster, "FP.State"=w229:T5)
            n89 = Not Equal?(x=w229, y=w227) -> (x != y?=w228:bool)
            n90 = case shown="True" w228 {
              tunnel: [w238 w239] -> w234
              tunnel: w231 -> [w237 w239]
              tunnel: w230 -> [w236 _]
              tunnel: w227 -> [w235 _]
              frame True {
                n91 = invoke class="VI" method="FP.Open"(reference=w236, error in=w237, "State"=w235) -> (error out=w238:errorcluster)  [unwired: 2 in, 4 out]
              }
              frame False {
              }
            }
          }
          frame "Maximize", "Maximized" {
            w240 = T5."Maximized" ("State")
            n92 = property class="VI"(reference=w246, error in=w245) -> (reference out=w243:refnum<vi>, error out=w244:errorcluster, "FP.State"=w242:T5)
            n93 = Not Equal?(x=w242, y=w240) -> (x != y?=w241:bool)
            n94 = case shown="True" w241 {
              tunnel: [w251 w252] -> w247
              tunnel: w244 -> [w250 w252]
              tunnel: w243 -> [w249 _]
              tunnel: w240 -> [w248 _]
              frame True {
                n95 = invoke class="VI" method="FP.Open"(reference=w249, error in=w250, "State"=w248) -> (error out=w251:errorcluster)  [unwired: 2 in, 4 out]
              }
              frame False {
              }
            }
          }
        }
        n96 = call <vilib>:"Add State(s) to Queue__JKI_lib_State_Machine.vi"("State(s) in (\"\")"=w187) -> ("States Out"=w186:string)  [unwired: 14 in]
      }
      frame "---------- Macro ----------" {
        # "Do not put any code in this frame.\n(It is a separator no-op. You can make a copy of this frame to create a new Macro frame)"
        n97 = call <vilib>:"Add State(s) to Queue__JKI_lib_State_Machine.vi"("State(s) in (\"\")"=w256) -> ("States Out"=w255:string)  [unwired: 14 in]
      }
      frame "Macro: Initialize" {
        w257 = "Data: Initialize\nInitialize Core Data\nReset Settings from UI\nUI: Initialize\nUI: Front Panel State >> Open\nError Handler"  # Data: Initialize Initialize Core Data Reset Settings from UI UI: Initialize UI: Front Panel State >> Open Error Handler
        # "Initialization Macro\n(This is called once, when the VI starts)"
        n98 = call <vilib>:"Add State(s) to Queue__JKI_lib_State_Machine.vi"("State(s) in Front (\"\")"=w257, "State(s) in (\"\")"=w261) -> ("States Out"=w260:string)  [unwired: 13 in]
      }
      frame "Macro: Exit" {
        # "Exit Macro\n(This is called once, when the VI exits)"
        n99 = Unbundle By Name(w268) -> ("Core.Close Panel on Exit?"=w267:bool)
        n100 = Select(t="UI: Front Panel State >> Close", s=w267, f="") -> (s? t:f=w264:string)
        n101 = call <vilib>:"Add State(s) to Queue__JKI_lib_State_Machine.vi"("State(s) in (\"\")"=w264, "State(s) at Back (\"\")"="Data: Cleanup\nExit") -> ("States Out"=w262:string)  [unwired: 13 in]
        n102 = call <vilib>:"Add State(s) to Queue__JKI_lib_State_Machine.vi"("State(s) in Front (\"\")"=w262, "State(s) in (\"\")"=w271) -> ("States Out"=w270:string)  [unwired: 13 in]
      }
      frame "---------- Steps ----------" {
        # "Template Separator\n(You can make a copy of, or modify, this frame)"
        n103 = call <vilib>:"Add State(s) to Queue__JKI_lib_State_Machine.vi"("State(s) in (\"\")"=w275) -> ("States Out"=w274:string)  [unwired: 14 in]
      }
      frame "Steps: Get Athlete Details" {
        # "Do not delete, rename, or modify this frame.\n(this is used to determine panel behavior on exit)"
        n104 = Unbundle By Name(w283) -> ("Strava"=w277:refnum<class "Strava curl.lvclass">)
        n105 = call-dynamic "Get Authenticated Athlete.vi"("error in (no error)"=w276, "Strava curl in"=w277) -> ("error out"=w280:errorcluster, "Response"=w281:string, "Strava curl out"=w282:refnum<class "Strava curl.lvclass">)  [unwired: 7 in]
        n106 = call <userlib>:"JSON Pretty Print.vi"("error in"=w280, "JSON String"=w281) -> ("error out"=w279:errorcluster, "JSON Pretty Print Format"=w278:string)  [unwired: 8 in]
        n107 = Bundle By Name(cluster=w283, "Strava"=w282) -> (w284:T8)
        n108 = call <vilib>:"Add State(s) to Queue__JKI_lib_State_Machine.vi"("State(s) in (\"\")"=w286) -> ("States Out"=w285:string)  [unwired: 14 in]
      }
      frame "Steps: Load Club Activity from Strava" {
        # "Your code here.\n(You can make a copy of, or modify, this frame)"
        n109 = Unbundle By Name(w305) -> ("Strava"=w304:refnum<class "Strava curl.lvclass">, "Data Manager"=w298:refnum<class "Data Manager.lvclass">)
        n110 = call-dynamic "Get Club Activities.vi"("error in (no error)"=w303, "Strava in"=w304) -> ("error out"=w297:errorcluster, "Response"=w299:string, "Strava out"=w300:refnum<class "Strava curl.lvclass">)  [unwired: 7 in]
        n111 = call-dynamic "Parse New Activities.vi"("error in (no error)"=w297, "Club Activities JSON"=w299, "Data Manager in"=w298) -> ("error out"=w296:errorcluster, "History"=w295:T7, "Strava Club Activities"=w288:T10[], "Data Manager out"=w292:refnum<class "Data Manager.lvclass">)  [unwired: 5 in]
        n112 = call-dynamic "Read Athlete Profile Map.vi"("Data Manager in"=w292) -> ("Athlete Profile Map"=w293:map{T3, T4})  [unwired: 8 in, 2 out]
        n113 = Array Size(array=w288) -> (size(s)=w287:i32)
        n114 = local write "Athlete Profile Map"(w293) -> ()
        n115 = global write "Globals.vi" "Data Manager"(w292) -> ()
        n116 = Bundle By Name(cluster=w305, "Strava"=w300, "Data Manager"=w292) -> (w302:T8)
        n117 = call <userlib>:"JSON Pretty Print.vi"("error in"=w296, "JSON String"=w299) -> ("error out"=w301:errorcluster, "JSON Pretty Print Format"=w291:string)  [unwired: 8 in]
        n118 = Unbundle By Name(w295) -> ("All Records"=→"History":string[][])
        n119 = Format Into String(format string="Added %d Records\n%s", w287, w291) -> (resulting string=w290:string)  [unwired: 2 in, 1 out]
        n120 = call <vilib>:"Add State(s) to Queue__JKI_lib_State_Machine.vi"("State(s) in (\"\")"=w307) -> ("States Out"=w306:string)  [unwired: 14 in]
      }
      frame "Steps: Load Club Members" {
        # "Your code here.\n(You can make a copy of, or modify, this frame)"
        n121 = Unbundle By Name(w320) -> ("Strava"=w319:refnum<class "Strava curl.lvclass">, "Data Manager"=w311:refnum<class "Data Manager.lvclass">)
        n122 = call-dynamic "Get Club Members.vi"("error in (no error)"=w318, "Strava in"=w319) -> ("error out"=w309:errorcluster, "Response"=w312:string, "Strava out"=w314:refnum<class "Strava curl.lvclass">)  [unwired: 7 in]
        n123 = call-dynamic "Parse New Members.vi"("error in (no error)"=w309, "Club Members JSON"=w312, "Data Manager in"=w311) -> ("error out"=w308:errorcluster, "Data Manager out"=w310:refnum<class "Data Manager.lvclass">)  [unwired: 7 in]
        n124 = call-dynamic "Read Athlete Profile Map.vi"("Data Manager in"=w310) -> ("Athlete Profile Map"=w313:map{T3, T4})  [unwired: 8 in, 2 out]
        n125 = local write "Athlete Profile Map"(w313) -> ()
        n126 = Bundle By Name(cluster=w320, "Strava"=w314, "Data Manager"=w310) -> (w317:T8)
        n127 = call <userlib>:"JSON Pretty Print.vi"("error in"=w308, "JSON String"=w312) -> ("error out"=w316:errorcluster, "JSON Pretty Print Format"=w315:string)  [unwired: 8 in]
        n128 = call <vilib>:"Add State(s) to Queue__JKI_lib_State_Machine.vi"("State(s) in (\"\")"=w322) -> ("States Out"=w321:string)  [unwired: 14 in]
      }
      frame "Steps: Run SQL" {
        # "Your code here.\n(You can make a copy of, or modify, this frame)"
        n129 = Unbundle By Name(w333) -> ("Data Manager"=w331:refnum<class "Data Manager.lvclass">)
        n130 = call-dynamic "Run SQL.vi"("error in (no error)"=w329, "SQL"="SQL", "Data Manager in"=w331) -> ("error out"=w330:errorcluster, "Result Set"=→"Return":string[][], "Column Names"=w328:string[], "Data Manager out"=w326:refnum<class "Data Manager.lvclass">)  [unwired: 5 in]
        n131 = property on="Return" class="Tbl (strict)"("Column Headers[]"=w328) -> ()  [unwired: 2 in, 2 out]
        n132 = call <userlib>:"JSON Pretty Print.vi"("error in"=w330, "JSON String"="SQL") -> ("error out"=w325:errorcluster, "JSON Pretty Print Format"=w323:string)  [unwired: 8 in]
        n133 = Bundle By Name(cluster=w333, "Data Manager"=w326) -> (w332:T8)
        n134 = call <vilib>:"Add State(s) to Queue__JKI_lib_State_Machine.vi"("State(s) in (\"\")"=w335) -> ("States Out"=w334:string)  [unwired: 14 in]
      }
      frame "Steps: Export Image to Twitter" {
        # "Select Distinct Athlete, Sum(Distance_m/1000) AS Distance, Team from Activities \nWhere Valid = 1 \nGroup By Athlete\nOrder by Distance desc"
        # "Your code here.\n(You can make a copy of, or modify, this frame)"
        n135 = call "Leaderboard export.vi"("current time"="Date for Daily Gains", "path to PNG file"="path to PNG file") -> ("error out"=w340:errorcluster, "path"=w339:path)  [unwired: 8 in]
        n136 = case shown="No Error" w340 {
          selector: w340 -> [_ w347]
          tunnel: w339 -> [w346 _]
          tunnel: [w345 w347] -> w338
          frame No Error {
            n137 = call "Tweet with Image.vi"("Picture File (PNG, JPG, GIF)"=w346, "Tweet"="Tweet") -> ("error out"=w345:errorcluster)  [unwired: 9 in]
          }
          frame Error {
          }
        }
        n138 = call <vilib>:"Add State(s) to Queue__JKI_lib_State_Machine.vi"("State(s) in (\"\")"=w343) -> ("States Out"=w342:string)  [unwired: 14 in]
      }
    }
    n139 = call "Add Status.vi"("i"=w5, "New Status"=w4) -> ("Status history"=→"Status":string)  [unwired: 9 in]
  }
